vi "FuzzyEx Pattern Recognition.vi"() -> ()   [LabVIEW 2023]
doc: "This example illustrates how to use fuzzy logic to detect materials parts based on its shape."
uses:
  <vilib>/addons/Fuzzy Logic/TypeDefs/FL System.ctl
  <vilib>/addons/Fuzzy Logic/TypeDefs/FL Variable.ctl
  <vilib>/addons/Fuzzy Logic/TypeDefs/FL Membership Function.ctl
  <vilib>/addons/Fuzzy Logic/TypeDefs/FL Membership Function Shape.ctl
  <vilib>/addons/Fuzzy Logic/TypeDefs/FL Rule.ctl
  <vilib>/addons/Fuzzy Logic/TypeDefs/FL Antecedent.ctl
  <vilib>/addons/Fuzzy Logic/TypeDefs/FL Modifier.ctl
  <vilib>/addons/Fuzzy Logic/TypeDefs/FL Antecedent Connective.ctl
  <vilib>/addons/Fuzzy Logic/TypeDefs/FL Consequent.ctl
  <vilib>/addons/Fuzzy Logic/TypeDefs/FL Consequent Implication.ctl
  <vilib>/addons/Fuzzy Logic/TypeDefs/FL Defuzzification.ctl
  <vilib>/addons/Fuzzy Logic/TypeDefs/FL Interpolating polynomials.ctl
  <vilib>/addons/Fuzzy Logic/FL Fuzzy Controller (MISO).vi
  <vilib>/addons/Fuzzy Logic/NI_Fuzzy_Logic_API.lvlib
panel:
  out "fuzzy system out":T1={"input variables"=[{"name"="Up scanner 1", "range"=[-0.5, 1.5, -0.5, 1.5], "MFs"=[{"name"="Far", "shape"=1, "points"=[-0.5, -0.5, 0.2, 0.5], "color"=0, "user-defined shape index"=0}, {"name"="Medium", "shape"=0, "points"=[0.2, 0.5, 0.8], "color"=56363, "user-defined shape index"=0}, {"name"="Near", "shape"=1, "points"=[0.5, 0.8, 1.5, 1.5], "color"=0, "user-defined shape index"=0}]}, {"name"="Up scanner 2", "range"=[-0.5, 1.5, -0.5, 1.5], "MFs"=[{"name"="Far", "shape"=1, "points"=[-0.5, -0.5, 0.2, 0.5], "color"=0, "user-defined shape index"=0}, {"name"="Medium", "shape"=0, "points"=[0.2, 0.5, 0.8], "color"=56363, "user-defined shape index"=0}, {"name"="Near", "shape"=1, "points"=[0.5, 0.8, 1.5, 1.5], "color"=0, "user-defined shape index"=0}]}, {"name"="Up scanner 3", "range"=[-0.5, 1.5, -0.5, 1.5], "MFs"=[{"name"="Far", "shape"=1, "points"=[-0.5, -0.5, 0.2, 0.5], "color"=0, "user-defined shape index"=0}, {"name"="Medium", "shape"=0, "points"=[0.2, 0.5, 0.8], "color"=56363, "user-defined shape index"=0}, {"name"="Near", "shape"=1, "points"=[0.5, 0.8, 1.5, 1.5], "color"=0, "user-defined shape index"=0}]}, {"name"="Down scanner 1", "range"=[-1.5, 0.5, -1.5, 0.5], "MFs"=[{"name"="Near", "shape"=1, "points"=[-1.5, -1.5, -0.8, -0.5], "color"=0, "user-defined shape index"=0}, {"name"="Medium", "shape"=0, "points"=[-0.8, -0.5, -0.2], "color"=16711680, "user-defined shape index"=0}, {"name"="Far", "shape"=1, "points"=[-0.5, -0.19999999999999996, 0.5, 0.5], "color"=0, "user-defined shape index"=0}]}, {"name"="Down scanner 2", "range"=[-1.5, 0.5, -1.5, 0.5], "MFs"=[{"name"="Near", "shape"=1, "points"=[-1.5, -1.5, -0.8, -0.5], "color"=0, "user-defined shape index"=0}, {"name"="Medium", "shape"=0, "points"=[-0.8, -0.5, -0.2], "color"=16711680, "user-defined shape index"=0}, {"name"="Far", "shape"=1, "points"=[-0.5, -0.2, 0.5, 0.5], "color"=0, "user-defined shape index"=0}]}, {"name"="Down scanner 3", "range"=[-1.5, 0.5, -1.5, 0.5], "MFs"=[{"name"="Near", "shape"=1, "points"=[-1.5, -1.5, -0.8, -0.5], "color"=0, "user-defined shape index"=0}, {"name"="Medium", "shape"=0, "points"=[-0.8, -0.5, -0.2], "color"=16711680, "user-defined shape index"=0}, {"name"="Far", "shape"=1, "points"=[-0.5, -0.2, 0.5, 0.5], "color"=0, "user-defined shape index"=0}]}], "output variables"=[{"name"="Part", "range"=[0.0, 6.0, 0.0, 6.0], "MFs"=[{"name"="Unknown", "shape"=0, "points"=[0.0, 0.0, 1.0], "color"=0, "user-defined shape index"=0}, {"name"="Square", "shape"=0, "points"=[0.0, 1.0, 2.0], "color"=1195007, "user-defined shape index"=0}, {"name"="Left trapezoid", "shape"=0, "points"=[1.0, 2.0, 3.0], "color"=2410496, "user-defined shape index"=0}, {"name"="Right trapezoid", "shape"=0, "points"=[2.0, 3.0, 4.0], "color"=11861920, "user-defined shape index"=0}, {"name"="Left triangle", "shape"=0, "points"=[3.0, 4.0, 5.0], "color"=11796480, "user-defined shape index"=0}, {"name"="Right triangle", "shape"=0, "points"=[4.0, 5.0, 6.0], "color"=16714752, "user-defined shape index"=0}, {"name"="Hexagon", "shape"=0, "points"=[5.0, 6.0, 6.0], "color"=16711934, "user-defined shape index"=0}]}], "rules"=[{"antecedents"=[{"Var Index"=0, "MF Index"=0, "Cond"=0}, {"Var Index"=1, "MF Index"=0, "Cond"=0}, {"Var Index"=2, "MF Index"=0, "Cond"=0}, {"Var Index"=3, "MF Index"=2, "Cond"=0}, {"Var Index"=4, "MF Index"=2, "Cond"=0}, {"Var Index"=5, "MF Index"=2, "Cond"=0}], "antecedent connective"=0, "consequents"=[{"Var Index"=0, "MF Index"=0, "Cond"=0}], "consequent implication"=0, "degree of support"=1.0}, {"antecedents"=[{"Var Index"=0, "MF Index"=2, "Cond"=0}, {"Var Index"=1, "MF Index"=2, "Cond"=0}, {"Var Index"=2, "MF Index"=2, "Cond"=0}, {"Var Index"=3, "MF Index"=0, "Cond"=0}, {"Var Index"=4, "MF Index"=0, "Cond"=0}, {"Var Index"=5, "MF Index"=0, "Cond"=0}], "antecedent connective"=0, "consequents"=[{"Var Index"=0, "MF Index"=1, "Cond"=0}], "consequent implication"=0, "degree of support"=1.0}, {"antecedents"=[{"Var Index"=0, "MF Index"=2, "Cond"=0}, {"Var Index"=1, "MF Index"=1, "Cond"=0}, {"Var Index"=2, "MF Index"=0, "Cond"=0}, {"Var Index"=3, "MF Index"=0, "Cond"=0}, {"Var Index"=4, "MF Index"=0, "Cond"=0}, {"Var Index"=5, "MF Index"=0, "Cond"=0}], "antecedent connective"=0, "consequents"=[{"Var Index"=0, "MF Index"=2, "Cond"=0}], "consequent implication"=0, "degree of support"=1.0}, {"antecedents"=[{"Var Index"=0, "MF Index"=0, "Cond"=0}, {"Var Index"=1, "MF Index"=1, "Cond"=0}, {"Var Index"=2, "MF Index"=2, "Cond"=0}, {"Var Index"=3, "MF Index"=0, "Cond"=0}, {"Var Index"=4, "MF Index"=0, "Cond"=0}, {"Var Index"=5, "MF Index"=0, "Cond"=0}], "antecedent connective"=0, "consequents"=[{"Var Index"=0, "MF Index"=3, "Cond"=0}], "consequent implication"=0, "degree of support"=1.0}, {"antecedents"=[{"Var Index"=0, "MF Index"=0, "Cond"=0}, {"Var Index"=1, "MF Index"=1, "Cond"=0}, {"Var Index"=2, "MF Index"=2, "Cond"=0}, {"Var Index"=3, "MF Index"=2, "Cond"=0}, {"Var Index"=4, "MF Index"=1, "Cond"=0}, {"Var Index"=5, "MF Index"=0, "Cond"=0}], "antecedent connective"=0, "consequents"=[{"Var Index"=0, "MF Index"=4, "Cond"=0}], "consequent implication"=0, "degree of support"=1.0}, {"antecedents"=[{"Var Index"=0, "MF Index"=2, "Cond"=0}, {"Var Index"=1, "MF Index"=1, "Cond"=0}, {"Var Index"=2, "MF Index"=0, "Cond"=0}, {"Var Index"=3, "MF Index"=0, "Cond"=0}, {"Var Index"=4, "MF Index"=1, "Cond"=0}, {"Var Index"=5, "MF Index"=2, "Cond"=0}], "antecedent connective"=0, "consequents"=[{"Var Index"=0, "MF Index"=5, "Cond"=0}], "consequent implication"=0, "degree of support"=1.0}, {"antecedents"=[{"Var Index"=0, "MF Index"=1, "Cond"=0}, {"Var Index"=1, "MF Index"=2, "Cond"=0}, {"Var Index"=2, "MF Index"=1, "Cond"=0}, {"Var Index"=3, "MF Index"=1, "Cond"=0}, {"Var Index"=4, "MF Index"=0, "Cond"=0}, {"Var Index"=5, "MF Index"=1, "Cond"=0}], "antecedent connective"=0, "consequents"=[{"Var Index"=0, "MF Index"=6, "Cond"=0}], "consequent implication"=0, "degree of support"=1.0}], "defuzzification method"=0, "description"="", "user MF interpolating polynomials"=[]} {"user MF interpolating polynomials"."coa_x(y) coeff" format="%.4g"; "user MF interpolating polynomials"."Area(y) coeff" format="%.4g"; "user MF interpolating polynomials"."X(y) coeff" format="%.4g"; "user MF interpolating polynomials"."Y(x) coeff" format="%.4g"; "user MF interpolating polynomials"."Y" format="%.4g"; "user MF interpolating polynomials"."X" format="%.4g"; "defuzzification method" items=["Center of Area", "Modified Center of Area", "Center of Sums", "Center of Maximum", "Mean of Maximum"]; "rules"."consequents"."Var Index" min=0; "rules"."consequents"."Cond" items=["=", "!="]; "rules"."consequents"."MF Index" min=0; "rules"."antecedents"."Var Index" min=0; "rules"."antecedents"."Cond" items=["=", "!="]; "rules"."antecedents"."MF Index" min=0; "rules"."consequent implication" items=["Minimum", "Product"]; "rules"."antecedent connective" items=["AND (Minimum)", "AND (Product)", "OR (Maximum)", "OR (Probabilistic)"]; "output variables"."MFs"."shape" items=["Triangle", "Trapezoid", "Singleton", "Sigmoid", "Gaussian", "User-Defined"]; "input variables"."MFs"."shape" items=["Triangle", "Trapezoid", "Singleton", "Sigmoid", "Gaussian", "User-Defined"]}
  out "Identified Part":u16(ring) items=["not detected", "Square", "Left Trapezoid", "Right Trapezoid", "Left Triangle", "Right Triangle", "Hexagon"]
  in  "Stop":bool
  out "Down Scanner":i32(slide) scale=0.0..200.0
  out "Up Scanner":i32(slide) scale=0.0..200.0
  out "Down Reading":dbl(slide)
  out "Up Reading":dbl(slide) scale=0.0..1.5
  in  "Part":u16(ring)
  in  "Noise Amplitude":dbl(knob) min=0.0 max=1.0 scale=0.0..0.5
  out "Scanner Data":cluster{"element":dbl, "element":dbl}(graph)
  in  "Delay":u32(knob)=5 min=1 max=100 step=1 scale=1.0..9.0
  # "Overview: This example illustrates how to use fuzzy logic to detect material  parts based on shape information (pattern matching).\nInstructions:\n1. Run the VI.\n2. Click the Part below to select the component to be scanned. Verify the Fuzzy Logic response in Identified Part.\n3. Increase the Noise Amplitude and verify that the noise doesn't modify the identification of the part.\n4. Click Stop to stop the VI."
  # "IF"
  # "THEN"
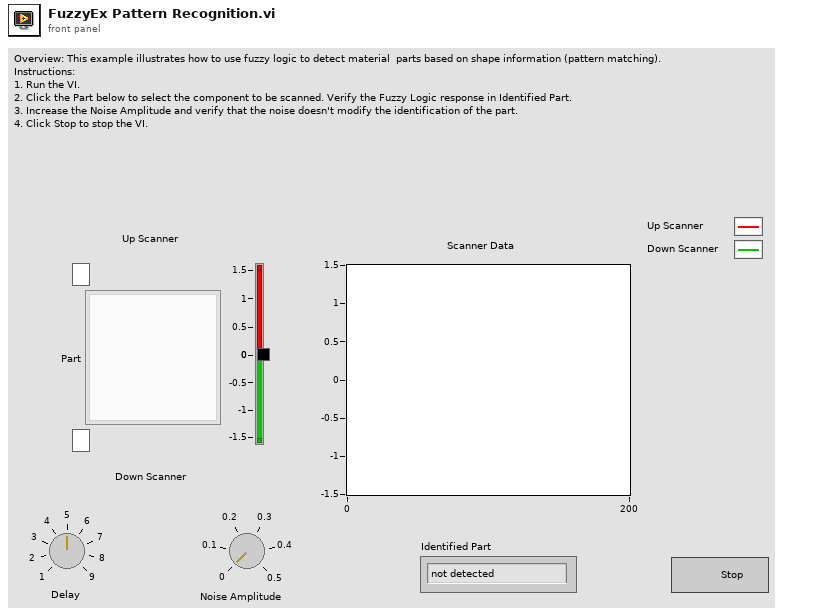
[diagram p1: front panel]
types:
  T1 = typedef "NI_Fuzzy_Logic_API.lvlib/FL System.ctl" = cluster{"input variables":T2[], "output variables":T2[], "rules":T5[], "defuzzification method":T11, "description":string, "user MF interpolating polynomials":T12[]}
  T2 = typedef "NI_Fuzzy_Logic_API.lvlib/FL Variable.ctl" = cluster{"name":string, "range":dbl[], "MFs":T3[]}
  T3 = typedef "NI_Fuzzy_Logic_API.lvlib/FL Membership Function.ctl" = cluster{"name":string, "shape":T4, "points":dbl[], "color":u32, "user-defined shape index":i32}
  T4 = typedef "NI_Fuzzy_Logic_API.lvlib/FL Membership Function Shape.ctl" = u16
  T5 = typedef "NI_Fuzzy_Logic_API.lvlib/FL Rule.ctl" = cluster{"antecedents":T6[], "antecedent connective":T8, "consequents":T9[], "consequent implication":T10, "degree of support":dbl}
  T6 = typedef "NI_Fuzzy_Logic_API.lvlib/FL Antecedent.ctl" = cluster{"Var Index":i32, "MF Index":i32, "Cond":T7}
  T7 = typedef "NI_Fuzzy_Logic_API.lvlib/FL Modifier.ctl" = u16
  T8 = typedef "NI_Fuzzy_Logic_API.lvlib/FL Antecedent Connective.ctl" = u16
  T9 = typedef "NI_Fuzzy_Logic_API.lvlib/FL Consequent.ctl" = cluster{"Var Index":i32, "MF Index":i32, "Cond":T7}
  T10 = typedef "NI_Fuzzy_Logic_API.lvlib/FL Consequent Implication.ctl" = u16
  T11 = typedef "NI_Fuzzy_Logic_API.lvlib/FL Defuzzification.ctl" = u16
  T12 = typedef "NI_Fuzzy_Logic_API.lvlib/FL Interpolating polynomials.ctl" = cluster{"X":dbl[], "Y":dbl[], "Y(x) coeff":dbl[][], "X(y) coeff":dbl[][], "Area(y) coeff":dbl[][], "coa_x(y) coeff":dbl[][]}
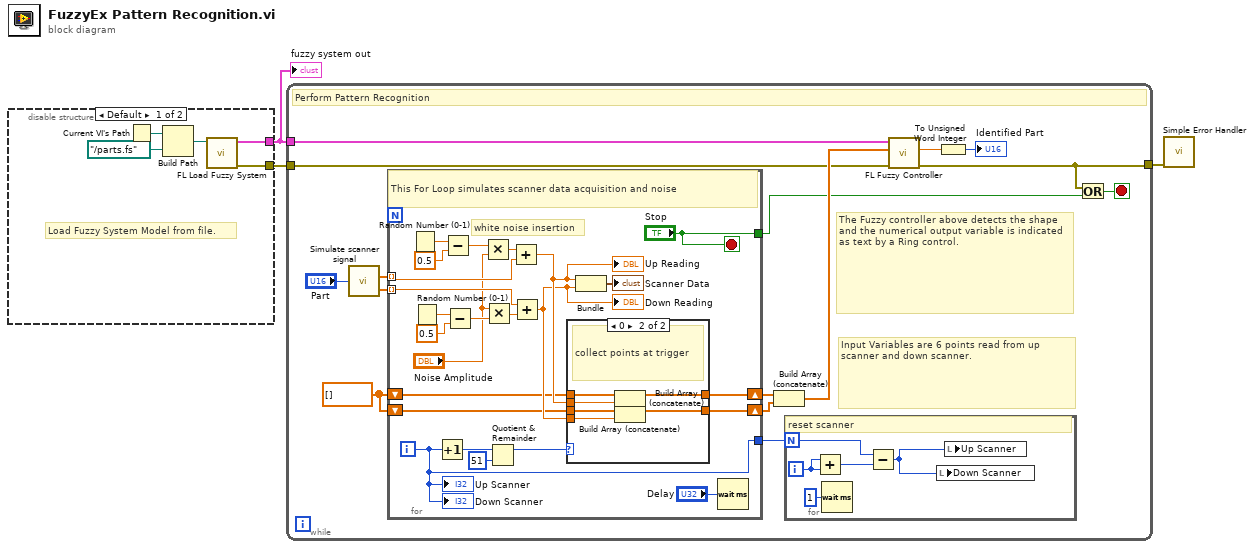
[diagram p0: block diagram]
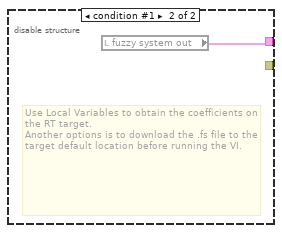
[diagram p2: hidden frame]
diagram:
  n1 = disable-structure shown="Default" {
    disable-tunnel: [w8 w9] -> w3
    disable-tunnel: [w4 _] -> w2
    frame condition #0 (active) {
      # "Load Fuzzy System Model from file."
      n2 = Current VI's Path() -> (path=w5:path)
      n3 = Build Path(base path=w5, name or relative path=path "../parts.fs") -> (appended path=w6:path)
      n4 = call <vilib>:"FL Load Fuzzy System.vi"("file path"=w6) -> ("error out"=w4:errorcluster, "fuzzy system out"=w8:T1)  [unwired: 1 in, 8 out]
    }
    frame condition #1 {
      # "Use Local Variables to obtain the coefficients on the RT target. \nAnother options is to download the .fs file to the target default location before running the VI."
      n5 = local read "fuzzy system out"() -> (w9:T1)
    }
  }
  "fuzzy system out" <- w3
  n6 = while {
    tunnel: w3 -> [w18]
    tunnel: w2 -> [w13]
    tunnel: [w11] -> w1
    stop <- w12 stop-if-true
    w21 = dbl[] []
    # "Input Variables are 6 points read from up scanner and down scanner."
    # "The Fuzzy controller above detects the shape and the numerical output variable is indicated as text by a Ring control."
    # "Perform Pattern Recognition"
    n7 = call "Simulate scanner signal.vi"("Form"="Part") -> ("Up Scanner"=w23:dbl[], "Down Scanner"=w22:dbl[])
    n8 = for {
      tunnel: w23 -> [w42] mode=indexing
      tunnel: w22 -> [w47] mode=indexing
      shift-right: [w39] -> w20
      shift-left: w21 -> [w36]
      shift-right: [w37] -> w19
      shift-left: w21 -> [w35]
      tunnel: [w31] -> w17
      tunnel: ["Stop"] -> w10
      i -> [w31]
      stop <- "Stop" stop-if-true
      # "white noise insertion"
      # "This For Loop simulates scanner data acquisition and noise"
      n9 = Random Number (0-1)() -> (number: 0 to 1=w44:dbl)
      n10 = Random Number (0-1)() -> (number: 0 to 1=w51:dbl)
      n11 = Increment(x=w31) -> (x+1=w34:i32)
      n12 = Subtract(x=w44, y=0.5) -> (x-y=w46:dbl)
      n13 = Subtract(x=w51, y=0.5) -> (x-y=w49:dbl)
      n14 = Multiply(x=w46, y="Noise Amplitude") -> (x*y=w43:dbl)
      n15 = Multiply(x="Noise Amplitude", y=w49) -> (x*y=w48:dbl)
      n16 = Quotient & Remainder(x=w34, y=51) -> (x-y*floor(x/y)=w32:i32)  [unwired: 1 out]
      n17 = Add(x=w43, y=w42) -> (x+y=w40:dbl)
      "Up Reading" <- w40
      n18 = Add(x=w47, y=w48) -> (x+y=w38:dbl)
      "Down Reading" <- w38
      n19 = case shown="0" w32 {
        tunnel: w40 -> [_ w61]
        tunnel: [w55 w60] -> w39
        tunnel: w38 -> [_ w59]
        tunnel: [w54 w58] -> w37
        tunnel: w36 -> [w55 w57]
        tunnel: w35 -> [w54 w56]
        frame Default {
        }
        frame 0 {
          # "collect points at trigger"
          n20 = Build Array (concatenate)(w57, w61) -> (w60:dbl[])
          n21 = Build Array (concatenate)(w56, w59) -> (w58:dbl[])
        }
      }
      n22 = Bundle(w40, w38) -> (→"Scanner Data":cluster{dbl, dbl})  [unwired: 1 out]
      n23 = Wait (ms)(milliseconds to wait="Delay") -> ()  [unwired: 1 out]
      "Up Scanner" <- w31
      "Down Scanner" <- w31
    }
    n24 = Build Array (concatenate)(w20, w19) -> (w15:dbl[])
    n25 = for {
      N: w17 -> [w25]
      i -> [w27]
      # "reset scanner"
      n26 = Add(x=w27, y=w27) -> (x+y=w28:i32)
      n27 = Wait (ms)(milliseconds to wait=u32 1) -> ()  [unwired: 1 out]
      n28 = Subtract(x=w25, y=w28) -> (x-y=w26:i32)
      n29 = local write "Down Scanner"(w26) -> ()
      n30 = local write "Up Scanner"(w26) -> ()
    }
    n31 = call-poly <vilib>:"FL Fuzzy Controller.vi"("error in (no error)"=w13, "input values"=w15, "fuzzy system in"=w18) -> ("error out"=w11:errorcluster, "output value"=w14:dbl)  [unwired: 7 out]
    n32 = To Unsigned Word Integer(number=w14) -> (unsigned 16bit integer=→"Identified Part":u16)
    n33 = Or(x=w11, y=w10) -> (x .or. y?=w12:bool)
  }
  n34 = call <vilib>:"Simple Error Handler.vi"("error in (no error)"=w1) -> ()  [unwired: 4 in, 5 out]
